vi "Run.vi"(8 "error in (no error)":errorcluster, 11 "Bank Account in":refnum<class "Bank Account.lvclass">) -> (0 "error out":errorcluster, 3 "Bank Account out":refnum<class "Bank Account.lvclass">)   [LabVIEW 2016, in "CLD Exam - ATM.lvlib" / "Bank Account.lvclass"]
uses:
  Bank Account.lvclass
  D:/Repos/Stream/software/Mediator/Classes/Mediated Actor/Mediated Actor.lvclass
  Mediator/Classes/Message Interface/Message Interface.lvclass
  Bank Account.lvclass/Bank Account.ctl
  Log/Application Log/Log Level.ctl
  Mediator/Classes/Message String/Message String.lvclass
  D:/Repos/Stream/software/Mediator/Classes/Message Interface/Message Interface.lvclass
  Mediator/Classes/Message Transport Queue/Message Transport Queue.lvclass
  D:/Repos/Stream/software/Mediator/Classes/Message Transport Interface/Message Transport Interface.lvclass
  Mediator/Classes/Mediated Actor/Mediated Actor.lvclass
  Log/Application Log/Application Log.lvclass
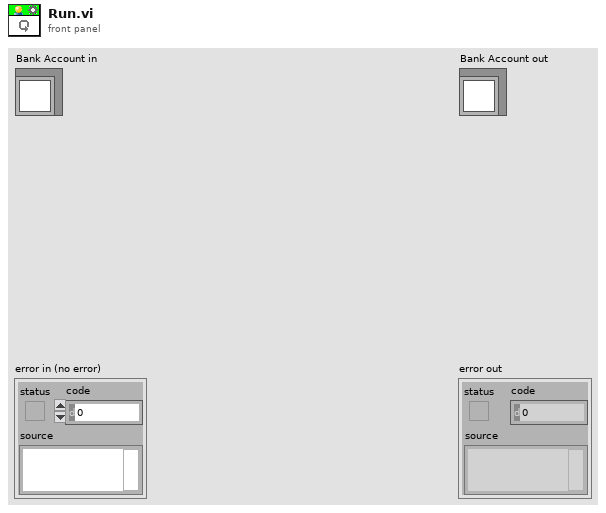
[diagram p1: front panel]
types:
  T1 = cluster{"System Exit":refnum<event-registration>, "Account Action Requested":refnum<event-registration>, "To Self":refnum<event-registration>}
  T2 = typedef "Stream Log.lvlib/Application Log.lvclass/Log Level.ctl" = enum16{"Imperative", "Major", "Minor", "Debug", "Off"}
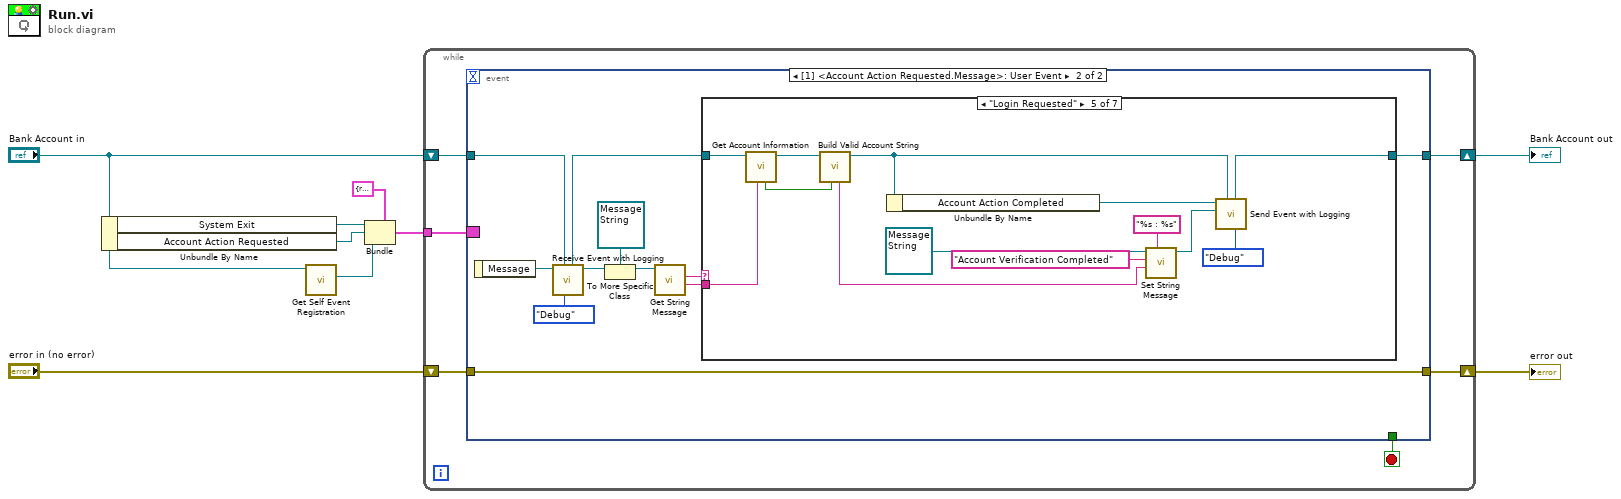
[diagram p0: block diagram]
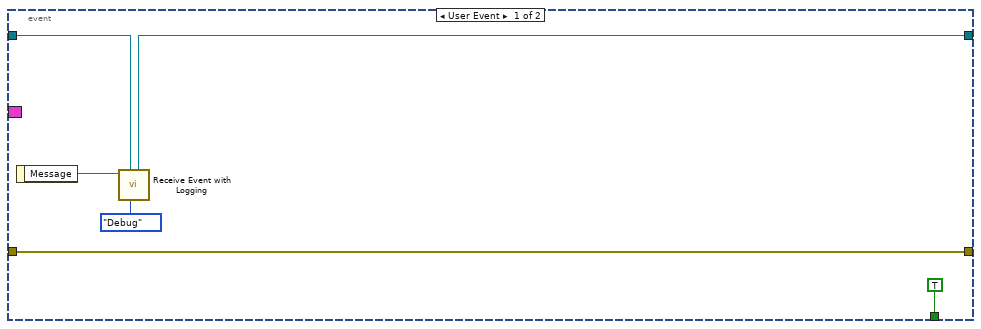
[diagram p2: hidden frame]
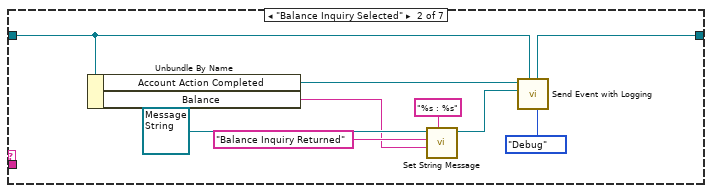
[diagram p4: hidden frame]
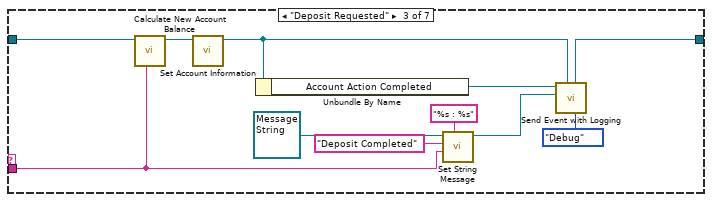
[diagram p5: hidden frame]
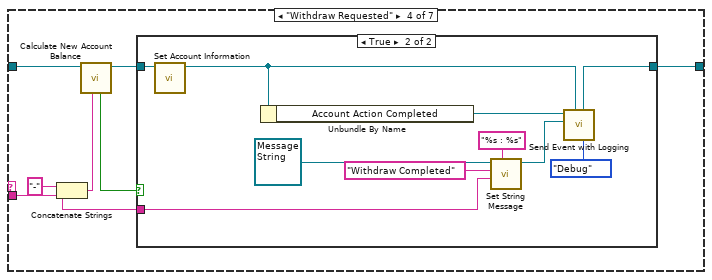
[diagram p6: hidden frame]
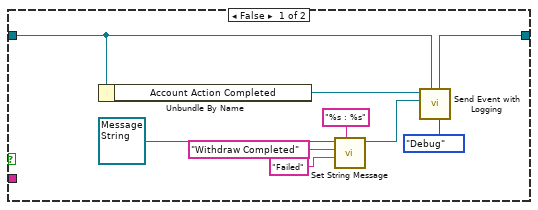
[diagram p7: hidden frame]
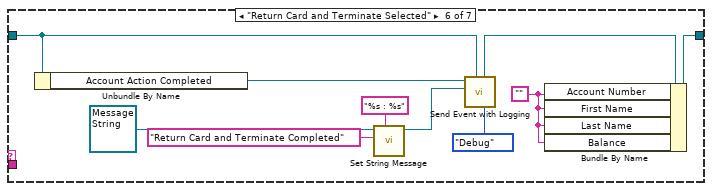
[diagram p8: hidden frame]
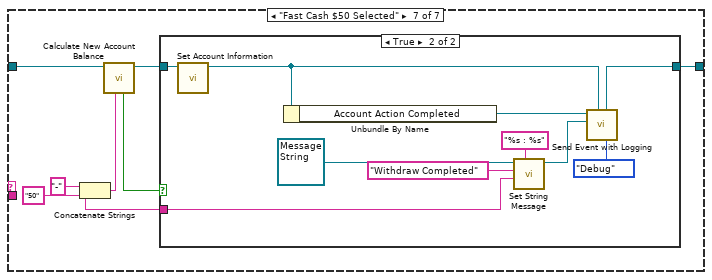
[diagram p9: hidden frame]
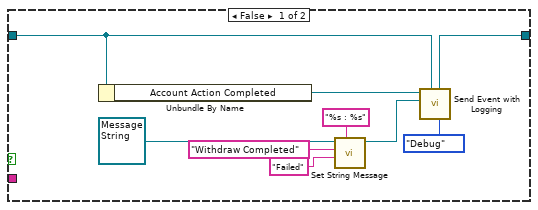
[diagram p10: hidden frame]
diagram:
  n1 = Unbundle By Name("Bank Account in") -> ("System Exit"=w5:refnum<event-registration>, "Account Action Requested"=w4:refnum<event-registration>)
  n2 = call "Get Self Event Registration.vi"("Mediated Actor in"="Bank Account in") -> ("Event Registration Refnum"=w3:refnum<event-registration>)  [unwired: 9 in, 1 out]
  n3 = Bundle(cluster=T1 {"System Exit"=refnum, "Account Action Requested"=refnum, "To Self"=refnum}, "System Exit"=w5, "Account Action Requested"=w4, "To Self"=w3) -> (w2:T1)
  n4 = while {
    shift-right: [w14] -> w9
    shift-left: "Bank Account in" -> [w15]
    shift-right: [w12] -> w7
    shift-left: "error in (no error)" -> [w13]
    tunnel: w2 -> [w11]
    stop <- w10 stop-if-true
    n5 = event shown="[1] <Account Action Requested.Message>: User Event" {
      selector: w11 -> [_ _]
      dyn-events: _ -> [_ _]
      timeout: _ -> [_ _]
      tunnel: w15 -> [w18 w24]
      tunnel: [w17 w29] -> w14
      tunnel: w13 -> [w21 w32]
      tunnel: [w21 w32] -> w12
      tunnel: [TRUE _] -> w10
      event User Event {
        n6 = event-data() -> ("Message"=w19:refnum<class "Message Interface.lvclass">)  [unwired: 1 in]
        n7 = call "Receive Event with Logging.vi"("Global Log Level"=Log_Level."Debug", "Mediated Actor in"=w18, "Message"=w19) -> ("Mediated Actor out"=w17:refnum<class "Bank Account.lvclass">)  [unwired: 5 in, 3 out]
      }
      event User Event {
        n8 = event-data() -> ("Message"=w26:refnum<class "Message Interface.lvclass">)  [unwired: 1 in]
        n9 = call "Receive Event with Logging.vi"("Global Log Level"=Log_Level."Debug", "Mediated Actor in"=w24, "Message"=w26) -> ("Message out"=w25:refnum<class "Message Interface.lvclass">, "Mediated Actor out"=w23:refnum<class "Bank Account.lvclass">)  [unwired: 5 in, 2 out]
        n10 = To More Specific Class(target class=refnum<class "Message String.lvclass"> refnum ("Message String in"), reference=w25) -> (specific class reference=w30:refnum<class "Message String.lvclass">)  [unwired: 1 in, 1 out]
        n11 = call "Get String Message.vi"("Message String in"=w30) -> ("Value"=w27:string, "Name"=w28:string)  [unwired: 7 in, 2 out]
        n12 = case shown="\"Login Requested\"" w28 {
          tunnel: w23 -> [w33 w36 w51 w60 w89 w96 w105]
          tunnel: [w33 w35 w44 w58 w85 w94 w104] -> w29
          tunnel: w27 -> [_ _ w50 w54 w88 _ _]
          frame Default {
          }
          frame "Balance Inquiry Selected" {
            n13 = Unbundle By Name(w36) -> ("Account Action Completed"=w38:refnum<class "Message Transport Queue.lvclass">, "Balance"=w40:string)
            n14 = call "Set String Message.vi"("Format"="%s : %s", "Value"=w40, "Name"="Balance Inquiry Returned", "Message String in"=refnum<class "Message String.lvclass"> refnum) -> ("Message String out"=w37:refnum<class "Message String.lvclass">)  [unwired: 6 in, 1 out]
            n15 = call "Send Event with Logging.vi"("Global Log Level"=Log_Level."Debug", "Mediated Actor in"=w36, "Message"=w37, "Message Transport Interface in"=w38) -> ("Mediated Actor out"=w35:refnum<class "Bank Account.lvclass">)  [unwired: 6 in, 1 out]
          }
          frame "Deposit Requested" {
            n16 = call "Calculate New Account Balance.vi"("Amount"=w50, "Bank Account in"=w51) -> ("Bank Account out"=w49:refnum<class "Bank Account.lvclass">)  [unwired: 7 in, 2 out]
            n17 = call "Set Account Information.vi"("Bank Account in"=w49) -> ("Bank Account out"=w45:refnum<class "Bank Account.lvclass">)  [unwired: 9 in, 1 out]
            n18 = Unbundle By Name(w45) -> ("Account Action Completed"=w47:refnum<class "Message Transport Queue.lvclass">)
            n19 = call "Set String Message.vi"("Format"="%s : %s", "Value"=w50, "Name"="Deposit Completed", "Message String in"=refnum<class "Message String.lvclass"> refnum) -> ("Message String out"=w46:refnum<class "Message String.lvclass">)  [unwired: 6 in, 1 out]
            n20 = call "Send Event with Logging.vi"("Global Log Level"=Log_Level."Debug", "Mediated Actor in"=w45, "Message"=w46, "Message Transport Interface in"=w47) -> ("Mediated Actor out"=w44:refnum<class "Bank Account.lvclass">)  [unwired: 6 in, 1 out]
          }
          frame "Withdraw Requested" {
            n21 = Concatenate Strings("-" ("string"), w54) -> (w56:string)
            n22 = call "Calculate New Account Balance.vi"("Amount"=w56, "Bank Account in"=w60) -> ("Bank Account out"=w59:refnum<class "Bank Account.lvclass">, "Sufficient Funds?"=w55:bool)  [unwired: 7 in, 1 out]
            n23 = case shown="True" w55 {
              tunnel: w59 -> [w63 w77]
              tunnel: [w62 w71] -> w58
              tunnel: w54 -> [_ w76]
              frame False {
                n24 = Unbundle By Name(w63) -> ("Account Action Completed"=w65:refnum<class "Message Transport Queue.lvclass">)
                n25 = call "Set String Message.vi"("Format"="%s : %s", "Value"="Failed", "Name"="Withdraw Completed", "Message String in"=refnum<class "Message String.lvclass"> refnum) -> ("Message String out"=w64:refnum<class "Message String.lvclass">)  [unwired: 6 in, 1 out]
                n26 = call "Send Event with Logging.vi"("Global Log Level"=Log_Level."Debug", "Mediated Actor in"=w63, "Message"=w64, "Message Transport Interface in"=w65) -> ("Mediated Actor out"=w62:refnum<class "Bank Account.lvclass">)  [unwired: 6 in, 1 out]
              }
              frame True {
                n27 = call "Set Account Information.vi"("Bank Account in"=w77) -> ("Bank Account out"=w72:refnum<class "Bank Account.lvclass">)  [unwired: 9 in, 1 out]
                n28 = Unbundle By Name(w72) -> ("Account Action Completed"=w74:refnum<class "Message Transport Queue.lvclass">)
                n29 = call "Set String Message.vi"("Format"="%s : %s", "Value"=w76, "Name"="Withdraw Completed", "Message String in"=refnum<class "Message String.lvclass"> refnum) -> ("Message String out"=w73:refnum<class "Message String.lvclass">)  [unwired: 6 in, 1 out]
                n30 = call "Send Event with Logging.vi"("Global Log Level"=Log_Level."Debug", "Mediated Actor in"=w72, "Message"=w73, "Message Transport Interface in"=w74) -> ("Mediated Actor out"=w71:refnum<class "Bank Account.lvclass">)  [unwired: 6 in, 1 out]
              }
            }
          }
          frame "Login Requested" {
            n31 = call "Get Account Information.vi"("Account Number"=w88, "Bank Account in"=w89) -> ("Bank Account out"=w83:refnum<class "Bank Account.lvclass">, "Account Verified?"=w81:bool)  [unwired: 7 in, 1 out]
            n32 = call "Build Valid Account String.vi"("Account Verified?"=w81, "Bank Account in"=w83) -> ("Bank Account out"=w82:refnum<class "Bank Account.lvclass">, "Value"=w80:string)  [unwired: 8 in]
            n33 = Unbundle By Name(w82) -> ("Account Action Completed"=w87:refnum<class "Message Transport Queue.lvclass">)
            n34 = call "Set String Message.vi"("Format"="%s : %s", "Value"=w80, "Name"="Account Verification Completed", "Message String in"=refnum<class "Message String.lvclass"> refnum) -> ("Message String out"=w86:refnum<class "Message String.lvclass">)  [unwired: 6 in, 1 out]
            n35 = call "Send Event with Logging.vi"("Global Log Level"=Log_Level."Debug", "Mediated Actor in"=w82, "Message"=w86, "Message Transport Interface in"=w87) -> ("Mediated Actor out"=w85:refnum<class "Bank Account.lvclass">)  [unwired: 6 in, 1 out]
          }
          frame "Return Card and Terminate Selected" {
            w93 = ""
            n36 = Unbundle By Name(w96) -> ("Account Action Completed"=w99:refnum<class "Message Transport Queue.lvclass">)
            n37 = call "Set String Message.vi"("Format"="%s : %s", "Name"="Return Card and Terminate Completed", "Message String in"=refnum<class "Message String.lvclass"> refnum) -> ("Message String out"=w98:refnum<class "Message String.lvclass">)  [unwired: 7 in, 1 out]
            n38 = call "Send Event with Logging.vi"("Global Log Level"=Log_Level."Debug", "Mediated Actor in"=w96, "Message"=w98, "Message Transport Interface in"=w99) -> ("Mediated Actor out"=w95:refnum<class "Bank Account.lvclass">)  [unwired: 6 in, 1 out]
            n39 = Bundle By Name(cluster=w95, "Account Number"=w93, "First Name"=w93, "Last Name"=w93, "Balance"=w93) -> (w94:refnum<class "Bank Account.lvclass">)
          }
          frame "Fast Cash $50 Selected" {
            w103 = "50" ("string")
            n40 = Concatenate Strings("-" ("string"), w103) -> (w107:string)
            n41 = call "Calculate New Account Balance.vi"("Amount"=w107, "Bank Account in"=w105) -> ("Bank Account out"=w109:refnum<class "Bank Account.lvclass">, "Sufficient Funds?"=w106:bool)  [unwired: 7 in, 1 out]
            n42 = case shown="True" w106 {
              tunnel: w109 -> [w112 w126]
              tunnel: [w111 w120] -> w104
              tunnel: w103 -> [_ w125]
              frame False {
                n43 = Unbundle By Name(w112) -> ("Account Action Completed"=w114:refnum<class "Message Transport Queue.lvclass">)
                n44 = call "Set String Message.vi"("Format"="%s : %s", "Value"="Failed", "Name"="Withdraw Completed", "Message String in"=refnum<class "Message String.lvclass"> refnum) -> ("Message String out"=w113:refnum<class "Message String.lvclass">)  [unwired: 6 in, 1 out]
                n45 = call "Send Event with Logging.vi"("Global Log Level"=Log_Level."Debug", "Mediated Actor in"=w112, "Message"=w113, "Message Transport Interface in"=w114) -> ("Mediated Actor out"=w111:refnum<class "Bank Account.lvclass">)  [unwired: 6 in, 1 out]
              }
              frame True {
                n46 = call "Set Account Information.vi"("Bank Account in"=w126) -> ("Bank Account out"=w121:refnum<class "Bank Account.lvclass">)  [unwired: 9 in, 1 out]
                n47 = Unbundle By Name(w121) -> ("Account Action Completed"=w123:refnum<class "Message Transport Queue.lvclass">)
                n48 = call "Set String Message.vi"("Format"="%s : %s", "Value"=w125, "Name"="Withdraw Completed", "Message String in"=refnum<class "Message String.lvclass"> refnum) -> ("Message String out"=w122:refnum<class "Message String.lvclass">)  [unwired: 6 in, 1 out]
                n49 = call "Send Event with Logging.vi"("Global Log Level"=Log_Level."Debug", "Mediated Actor in"=w121, "Message"=w122, "Message Transport Interface in"=w123) -> ("Mediated Actor out"=w120:refnum<class "Bank Account.lvclass">)  [unwired: 6 in, 1 out]
              }
            }
          }
        }
      }
    }
  }
  "error out" <- w7
  "Bank Account out" <- w9
